vi "Set Filter Parameters.vi"(5 "noise":i32, 6 "smooth":i32, 7 "accept":sgl, 9 "range":i32, 10 "sensitivity":sgl, 11 "width":i32) -> (3 "function return":u32)   [LabVIEW 2018, in "Copy of Andor SDK.lvlib"]
doc: "EXPNETTYPE unsigned int WINAPI SetFilterParameters(int width, float sensitivity, int range, float accept, int smooth, int noise);"
uses:
  Copy of Andor SDK.lvlib
  <userlib>/Andor SDK/ATMCD32D.dll
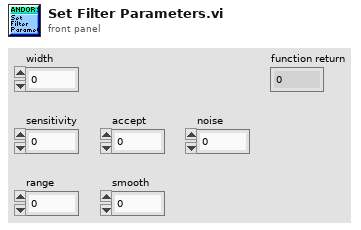
[diagram p1: front panel]
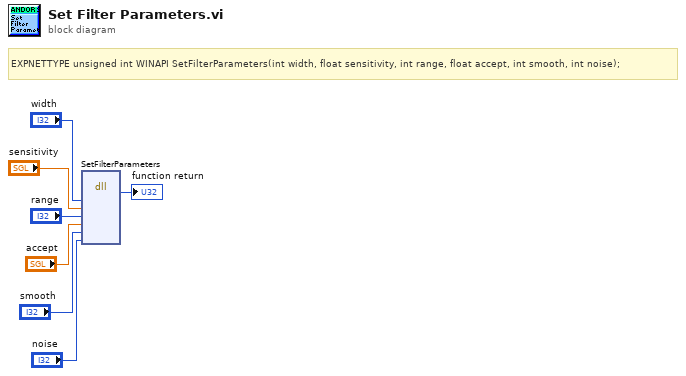
[diagram p0: block diagram]
diagram:
  # "EXPNETTYPE unsigned int WINAPI SetFilterParameters(int width, float sensitivity, int range, float accept, int smooth, int noise);"
  n1 = dll-call lib="C:/Program Files (x86)/National Instruments/LabVIEW 2018/user.lib/Andor SDK/ATMCD32D.*" fn="SetFilterParameters"("width"="width", "sensitivity"="sensitivity", "range"="range", "accept"="accept", "smooth"="smooth", "noise"="noise") -> (→"function return":u32)  [unwired: 9 in, 2 out]
